vi "Beam_Acceleration.vi"() -> ()   [LabVIEW 2018]
uses:
  InstrumentStatusLib/com.insstat.lvlib
panel:
  out "?":bool
  out "?":bool
  out "?":bool
  out "?":bool
  out "?":string
  out "?":string
  out "?":string
  out "?":string
  out "?":bool
  out "?":bool
  out "?":bool
  out "?":bool
  out "?":string
  out "?":string
  out "?":string
  out "?":string
  out "?":bool
  out "?":bool
  out "?":bool
  out "?":bool
  out "?":string
  out "?":string
  out "?":string
  out "?":string
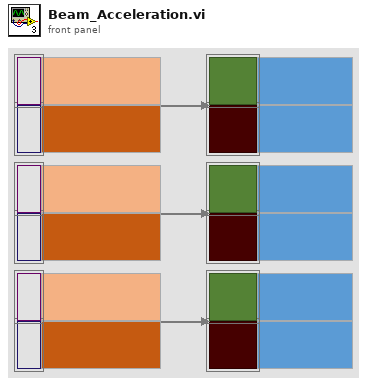
[diagram p1: front panel]
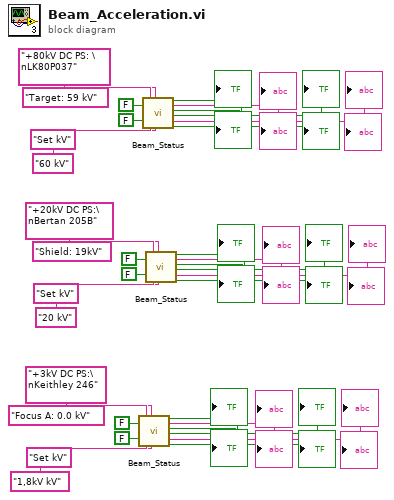
[diagram p0: block diagram]
diagram:
  n1 = call "Beam_Status.vi"("Power"=FALSE, "Activate"=FALSE, "String"="+3kV DC PS:\nKeithley 246", "String 3"="Set kV", "String 2"="Focus A: 0.0 kV", "String 4"="1,8kV kV") -> (10:→"?":string, 11:→"?":string, 12:→"?":string, 13:→"?":string, 14:→"?":bool, 16:→"?":bool, 17:→"?":bool, 19:→"?":bool)  [unwired: 6 in]
  n2 = call "Beam_Status.vi"("Power"=FALSE, "Activate"=FALSE, "String"="+80kV DC PS: \nLK80P037", "String 3"="Set kV", "String 2"="Target: 59 kV", "String 4"="60 kV") -> (10:→"?":string, 11:→"?":string, 12:→"?":string, 13:→"?":string, 14:→"?":bool, 16:→"?":bool, 17:→"?":bool, 19:→"?":bool)  [unwired: 6 in]
  n3 = call "Beam_Status.vi"("Power"=FALSE, "Activate"=FALSE, "String"="+20kV DC PS:\nBertan 205B", "String 3"="Set kV", "String 2"="Shield: 19kV", "String 4"="20 kV") -> (10:→"?":string, 11:→"?":string, 12:→"?":string, 13:→"?":string, 14:→"?":bool, 16:→"?":bool, 17:→"?":bool, 19:→"?":bool)  [unwired: 6 in]
